vi "AngleBetweenPoints.vi"(10 "Point 2":T1 {"North" format="%#_10f"; "East" format="%#_8f"}, 11 "Point 1":T1 {"North" format="%#_10f"; "East" format="%#_8f"}) -> (2 "Angle":dbl)   [LabVIEW 2013]
doc: "Takes in two UTM points and calculates the angle between them. The angle is in the standard reference frame."
uses:
  Data/TypeDefs/UTM Location.ctl
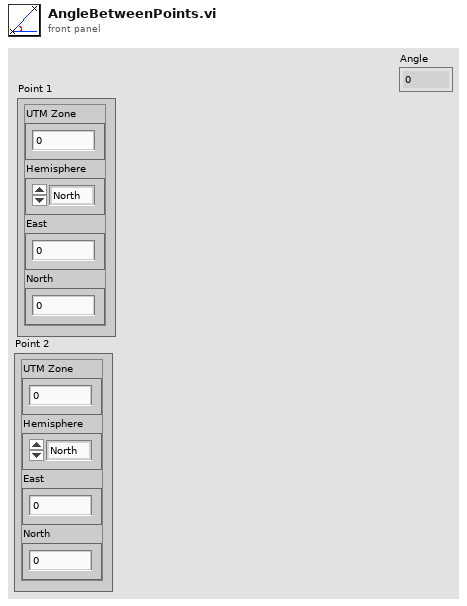
[diagram p1: front panel]
types:
  T1 = typedef "UTM Location.ctl" = cluster{"UTM Zone":dbl, "Hemisphere":enum16{"North", "South"}, "East":dbl, "North":dbl}
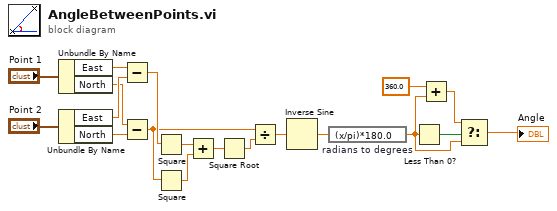
[diagram p0: block diagram]
diagram:
  n1 = Unbundle By Name("Point 1") -> ("East"=w17:dbl, "North"=w14:dbl)
  n2 = Unbundle By Name("Point 2") -> ("East"=w16:dbl, "North"=w15:dbl)
  n3 = Subtract(x=w17, y=w16) -> (x-y=w13:dbl)
  n4 = Subtract(x=w14, y=w15) -> (x-y=w8:dbl)
  n5 = Square(x=w13) -> (x^2=w12:dbl)
  n6 = Square(x=w8) -> (x^2=w11:dbl)
  n7 = Add(x=w12, y=w11) -> (x+y=w10:dbl)
  n8 = Square Root(x=w10) -> (sqrt(x)=w9:dbl)
  n9 = Divide(x=w8, y=w9) -> (x/y=w7:dbl)
  n10 = Inverse Sine(1:w7) -> (0:w6:dbl)
  n11 = expression code="(x/pi)*180.0" "radians to degrees"(w6) -> (w2:dbl)
  n12 = Less Than 0?(x=w2) -> (x < 0?=w5:bool)
  n13 = Add(x=360.0, y=w2) -> (x+y=w4:dbl)
  n14 = Select(t=w4, s=w5, f=w2) -> (s? t:f=→"Angle":dbl)
